vi "GET USER INFO.vi"(10 "USER/ITEM DATA TRANSFER IN":T3(array[cluster]), 11 "REFERENCES":T2) -> (3 "USER INFO OUT":T1)   [LabVIEW 2019]
uses:
  Controls/References Cluster.ctl
  Controls/Custom Calendar/Custom Calendar.xctl
  Controls/Table Data Types/User Data Type.ctl
  <vilib>/addons/database/Connection.llb/DB Tools Open Connec (String).vi
  <vilib>/addons/database/_DB Variant To Data/Database Variant To Data.xnode
  <vilib>/addons/database/NI_Database_API.lvlib
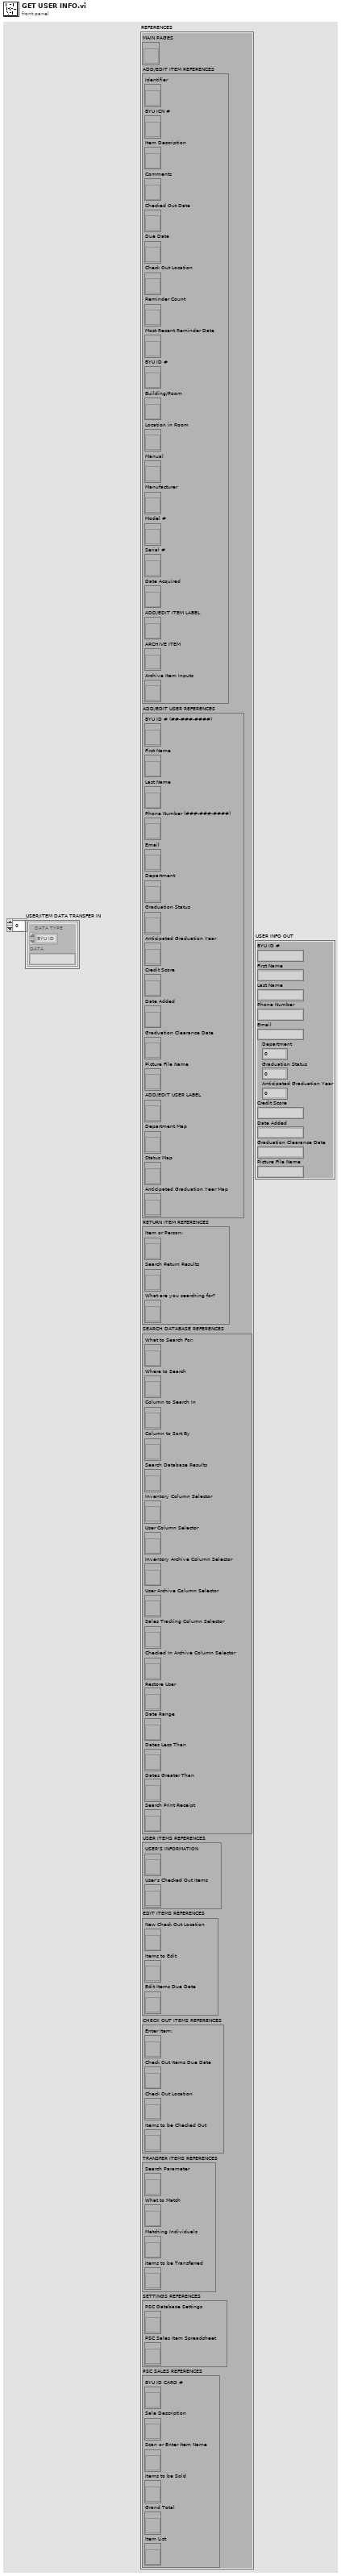
[diagram p1: front panel]
types:
  T1 = cluster{"BYU ID #":string, "First Name":string, "Last Name":string, "Phone Number":string, "Email":string, "Department":u16, "Graduation Status":u16, "Anticipated Graduation Year":u16, "Credit Score":string, "Date Added":string, "Graduation Clearance Date":string, "Picture File Name":string}
  T2 = typedef "References Cluster.ctl" = cluster{"MAIN PAGES":refnum<vi>, "ADD/EDIT ITEM REFERENCES":cluster{"Identifier":refnum<vi>, "BYU ICN #":refnum<vi>, "Item Description":refnum<vi>, "Comments":refnum<vi>, "Checked Out Date":refnum<vi>, "Due Date":refnum<vi>, "Check Out Location":refnum<vi>, "Reminder Count":refnum<vi>, "Most Recent Reminder Date":refnum<vi>, "BYU ID #":refnum<vi>, "Building/Room":refnum<vi>, "Location in Room":refnum<vi>, "Manual":refnum<vi>, "Manufacturer":refnum<vi>, "Model #":refnum<vi>, "Serial #":refnum<vi>, "Date Acquired":refnum<vi>, "ADD/EDIT ITEM LABEL":refnum<vi>, "ARCHIVE ITEM":refnum<vi>, "Archive Item Inputs":refnum<vi>}, "ADD/EDIT USER REFERENCES":cluster{"BYU ID # (##-###-####)":refnum<vi>, "First Name":refnum<vi>, "Last Name":refnum<vi>, "Phone Number (###-###-####)":refnum<vi>, "Email":refnum<vi>, "Department":refnum<vi>, "Graduation Status":refnum<vi>, "Anticipated Graduation Year":refnum<vi>, "Credit Score":refnum<vi>, "Date Added":refnum<vi>, "Graduation Clearance Date":refnum<vi>, "Picture File Name":refnum<vi>, "ADD/EDIT USER LABEL":refnum<vi>, "Department Map":refnum<vi>, "Status Map":refnum<vi>, "Anticipated Graduation Year Map":refnum<vi>}, "RETURN ITEM REFERENCES":cluster{"Item or Person:":refnum<vi>, "Search Return Results":refnum<vi>, "What are you searching for?":refnum<vi>}, "SEARCH DATABASE REFERENCES":cluster{"What to Search For:":refnum<vi>, "Where to Search":refnum<vi>, "Column to Search In":refnum<vi>, "Column to Sort By":refnum<vi>, "Search Database Results":refnum<vi>, "Inventory Column Selector":refnum<vi>, "User Column Selector":refnum<vi>, "Inventory Archive Column Selector":refnum<vi>, "User Archive Column Selector":refnum<vi>, "Sales Tracking Column Selector":refnum<vi>, "Checked In Archive Column Selector":refnum<vi>, "Restore User":refnum<vi>, "Date Range":refnum<vi>, "Dates Less Than":refnum<vi>, "Dates Greater Than":refnum<vi>, "Search Print Receipt":refnum<vi>}, "USER ITEMS REFERENCES":cluster{"USER'S INFORMATION":refnum<vi>, "User's Checked Out Items":refnum<vi>}, "EDIT ITEMS REFERENCES":cluster{"New Check Out Location":refnum<vi>, "Items to Edit":refnum<vi>, "Edit Items Due Date":refnum<vi>}, "CHECK OUT ITEMS REFERENCES":cluster{"Enter Item:":refnum<vi>, "Check Out Items Due Date":refnum<vi>, "Check Out Location":refnum<vi>, "Items to be Checked Out":refnum<vi>}, "TRANSFER ITEMS REFERENCES":cluster{"Search Parameter":refnum<vi>, "What to Match":refnum<vi>, "Matching Individuals":refnum<vi>, "Items to be Transferred":refnum<vi>}, "SETTINGS REFERENCES":cluster{"PSC Database Settings":refnum<vi>, "PSC Sales Item Spreadsheet":refnum<vi>}, "PSC SALES REFERENCES":cluster{"BYU ID CARD #":refnum<vi>, "Sale Description":refnum<vi>, "Scan or Enter Item Name":refnum<vi>, "Items to be Sold":refnum<vi>, "Grand Total":refnum<vi>, "Item List":refnum<vi>}}
  T3 = cluster{"DATA TYPE":enum16{"BYU ID", "ME#/IDENTIFIER", "BYU ICN"}, "DATA":string}[]
  T4 = typedef "User Data Type.ctl" = cluster{"BYU ID #":string, "First Name":string, "Last Name":string, "Phone Number":string, "Email":string, "Department":string, "Graduation Status":string, "Anticipated Graduation Year":string, "Credit Score":dbl, "Date Added":string, "Graduation Clearance Date":string, "Picture File Name":string}
  T5 = cluster{"BYU ID # (##-###-####)":refnum<vi>, "First Name":refnum<vi>, "Last Name":refnum<vi>, "Phone Number (###-###-####)":refnum<vi>, "Email":refnum<vi>, "Department":refnum<vi>, "Graduation Status":refnum<vi>, "Anticipated Graduation Year":refnum<vi>, "Credit Score":refnum<vi>, "Date Added":refnum<vi>, "Graduation Clearance Date":refnum<vi>, "Picture File Name":refnum<vi>, "ADD/EDIT USER LABEL":refnum<vi>, "Department Map":refnum<vi>, "Status Map":refnum<vi>, "Anticipated Graduation Year Map":refnum<vi>}
  T6 = cluster{"DATA TYPE":enum16{"BYU ID", "ME#/IDENTIFIER", "BYU ICN"}, "DATA":string}
  T7 = typedef "NI_Database_API.lvlib/Conn ObjectReference.ctl" = refnum<k1>
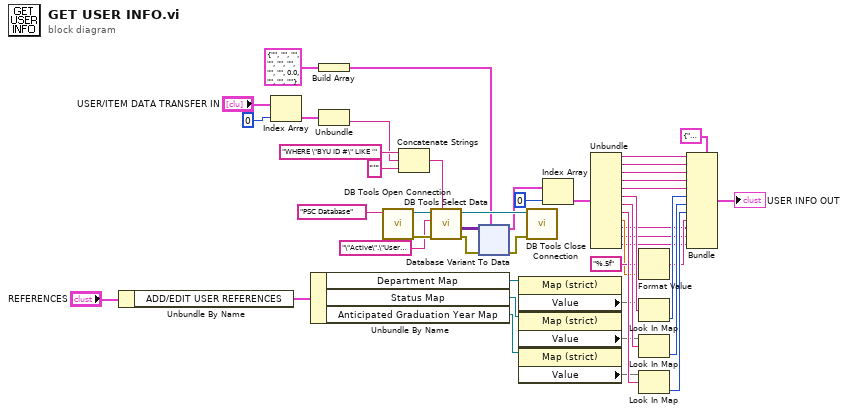
[diagram p0: block diagram]
diagram:
  n1 = Unbundle By Name("REFERENCES") -> ("ADD/EDIT USER REFERENCES"=w29:T5)
  n2 = Index Array(array="USER/ITEM DATA TRANSFER IN", index=0) -> (element=w46:T6)
  n3 = Unbundle By Name(w29) -> ("Department Map"=w28:refnum<vi>, "Status Map"=w27:refnum<vi>, "Anticipated Graduation Year Map"=w26:refnum<vi>)
  n4 = Build Array(T4 {"BYU ID #"="", "First Name"="", "Last Name"="", "Phone Number"="", "Email"="", "Department"="", "Graduation Status"="", "Anticipated Graduation Year"="", "Credit Score"=0.0, "Date Added"="", "Graduation Clearance Date"="", "Picture File Name"=""} ("Array")) -> (w9:T4[])
  n5 = Unbundle(w46) -> ("DATA"=w40:string)  [unwired: 1 out]
  n6 = call-poly <vilib>:"DB Tools Open Connection.vi"("connection information"="PSC Database") -> ("error out"=w44:errorcluster, "connection reference"=w45:T7)  [unwired: 7 in]
  n7 = Concatenate Strings("WHERE \"BYU ID #\" LIKE '" ("string"), w40, "'" ("string")) -> (w39:string)
  n8 = call <vilib>:"DB Tools Select Data.vi"("condition"=w39, "error in (no error)"=w44, "table"="\"Active\".\"Users\"", "connection reference"=w45) -> ("error out"=w37:errorcluster, "data"=w36:variant[][], "connection reference out"=w34:T7)  [unwired: 2 in]
  n9 = xnode "Database Variant To Data"("database variant"=w36, "error in (no error)"=w37, "type"=w9) -> ("data"=w33:T4[], "error out"=w35:errorcluster)
  n10 = property class="Map (strict)"(reference=w28) -> ("Value"=w20:map{string, i32})  [unwired: 1 in, 2 out]
  n11 = property class="Map (strict)"(reference=w27) -> ("Value"=w21:map{string, i32})  [unwired: 1 in, 2 out]
  n12 = property class="Map (strict)"(reference=w26) -> ("Value"=w22:map{string, i32})  [unwired: 1 in, 2 out]
  n13 = call <vilib>:"DB Tools Close Connection.vi"("error in (no error)"=w35, "connection reference"=w34) -> ()  [unwired: 5 in, 1 out]
  n14 = Index Array(array=w33, index=0) -> (element=w31:T4)
  n15 = Unbundle(w31) -> ("BYU ID #"=w19:string, "First Name"=w18:string, "Last Name"=w17:string, "Phone Number"=w16:string, "Email"=w15:string, "Department"=w23:string, "Graduation Status"=w25:string, "Anticipated Graduation Year"=w24:string, "Credit Score"=w7:dbl, "Date Added"=w3:string, "Graduation Clearance Date"=w2:string, "Picture File Name"=w1:string)
  n16 = Format Value(format string="%.5f", value (0)=w7) -> (output string=w6:string)  [unwired: 1 in]
  n17 = Look In Map(map=w20, key=w23) -> (value=w14:i32)  [unwired: 1 in, 1 out]
  n18 = Look In Map(map=w21, key=w25) -> (value=w12:i32)  [unwired: 1 in, 1 out]
  n19 = Look In Map(map=w22, key=w24) -> (value=w13:i32)  [unwired: 1 in, 1 out]
  n20 = Bundle(cluster=T1 {"BYU ID #"="", "First Name"="", "Last Name"="", "Phone Number"="", "Email"="", "Department"=0, "Graduation Status"=0, "Anticipated Graduation Year"=0, "Credit Score"="", "Date Added"="", "Graduation Clearance Date"="", "Picture File Name"=""} ("USER INFO OUT"), "BYU ID #"=w19, "First Name"=w18, "Last Name"=w17, "Phone Number"=w16, "Email"=w15, "Department"=w14, "Graduation Status"=w12, "Anticipated Graduation Year"=w13, "Credit Score"=w6, "Date Added"=w3, "Graduation Clearance Date"=w2, "Picture File Name"=w1) -> (→"USER INFO OUT":T1)
